vi "Get G-CLI Apps.vi"() -> ()   [LabVIEW 2020]
panel:
  in  "CopyClipboard":bool
  in  "OpenExplorer":bool
  out "GCLI Apps Path":path
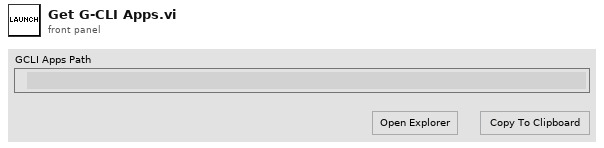
[diagram p1: front panel]
types:
  T1 = enum32{"Invalid", "Standard", "Closed", "Hidden", "Minimized", "Maximized"}
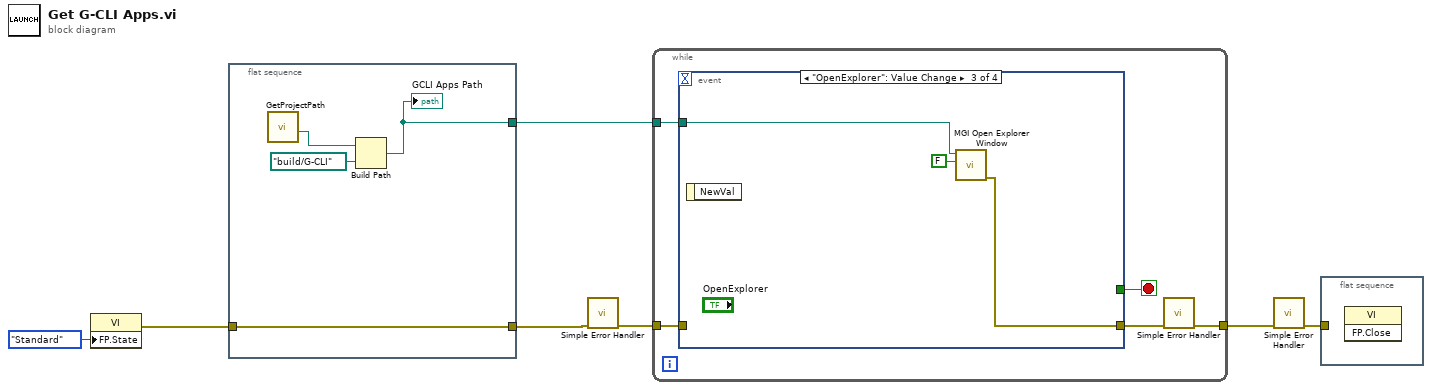
[diagram p0: block diagram]
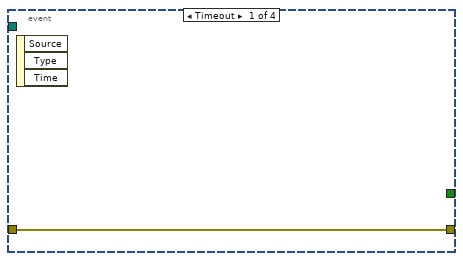
[diagram p2: hidden frame]
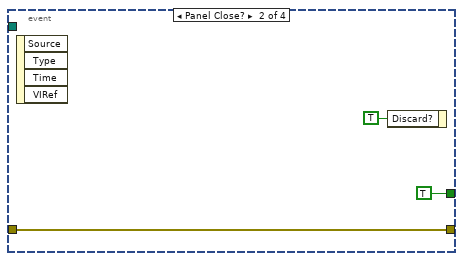
[diagram p3: hidden frame]
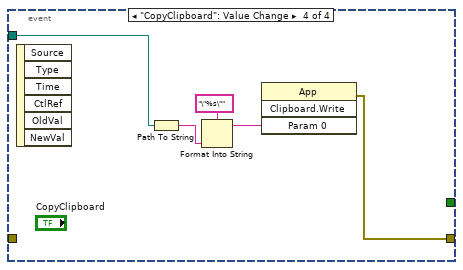
[diagram p4: hidden frame]
diagram:
  n1 = property class="VI"("FP.State"=T1."Standard" ("Front Panel Window:State")) -> (error out=w6:errorcluster)  [unwired: 2 in, 1 out]
  n2 = flat-sequence {
    tunnel: w6 -> [w9]
    tunnel: [w9] -> w3
    tunnel: [w8] -> w1
    frame #0 {
      n3 = call "GetProjectPath.vi"() -> ("ProjectRootPath"=w10:path)  [unwired: 10 in, 1 out]
      n4 = Build Path(base path=w10, name or relative path=path "build/G-CLI") -> (appended path=w8:path)
      "GCLI Apps Path" <- w8
    }
  }
  n5 = call <vilib>:"Simple Error Handler.vi"("error in (no error)"=w3) -> ("error out"=w5:errorcluster)  [unwired: 4 in, 4 out]
  n6 = while {
    tunnel: w5 -> [w15]
    tunnel: [w12] -> w4
    tunnel: w1 -> [w13]
    stop <- w16 stop-if-true
    n7 = event shown="[2] \"OpenExplorer\": Value Change" {
      selector: _ -> [_ _ _ _]
      dyn-events: _ -> [_ _ _ _]
      timeout: _ -> [_ _ _ _]
      tunnel: [_ TRUE _ _] -> w16
      tunnel: w15 -> [w17 w18 _ _]
      tunnel: [w17 w18 w21 w28] -> w14
      tunnel: w13 -> [_ _ w22 w27]
      event Timeout {
        n8 = event-data() -> ()  [unwired: 1 in, 3 out]
      }
      event Panel Close? {
        n9 = event-data() -> ()  [unwired: 1 in, 4 out]
        n10 = event-data("Discard?"=TRUE) -> ()  [unwired: 1 in, 1 out]
      }
      event "OpenExplorer": Value Change {
        n11 = event-data() -> ()  [unwired: 1 in, 1 out]
        n12 = call <userlib>:"MGI Open Explorer Window.vi"("Select Directory? (F: Open Directory)"=FALSE, "Directory or File"=w22) -> ("error out"=w21:errorcluster)  [unwired: 9 in]
      }
      event "CopyClipboard": Value Change {
        n13 = event-data() -> ()  [unwired: 1 in, 6 out]
        n14 = Path To String(path=w27) -> (string=w26:string)
        n15 = Format Into String(format string="\"%s\"", w26) -> (resulting string=w25:string)  [unwired: 2 in, 1 out]
        n16 = invoke class="App" method="Clipboard.Write"("Param 0"=w25) -> (error out=w28:errorcluster)  [unwired: 3 in, 3 out]
      }
    }
    n17 = call <vilib>:"Simple Error Handler.vi"("error in (no error)"=w14) -> ("error out"=w12:errorcluster)  [unwired: 4 in, 4 out]
  }
  n18 = call <vilib>:"Simple Error Handler.vi"("error in (no error)"=w4) -> ("error out"=w2:errorcluster)  [unwired: 4 in, 4 out]
  n19 = flat-sequence {
    tunnel: w2 -> [_]
    frame #0 {
      n20 = invoke class="VI" method="FP.Close"() -> ()  [unwired: 3 in, 3 out]
    }
  }
